vi "query_parts.vi"(8 "error in (no error)":errorcluster, 11 "DB Session ID":i32) -> (0 "error out":errorcluster, 1 "Parts":T1[](array[typedef]), 3 "DB Session ID out":i32)   [LabVIEW 2023, in "Database.lvlib"]
uses:
  Database.lvlib
  DB Part.ctl
  bin/Database.dll
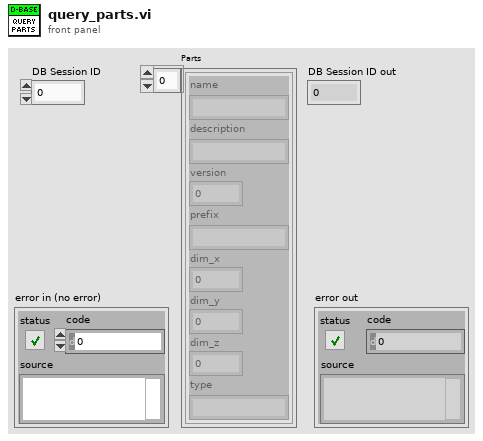
[diagram p1: front panel]
types:
  T1 = typedef "Database.lvlib/DB Part.ctl" = cluster{"name":string, "description":string, "version":i32, "prefix":string, "dim_x":sgl, "dim_y":sgl, "dim_z":sgl, "type":string}
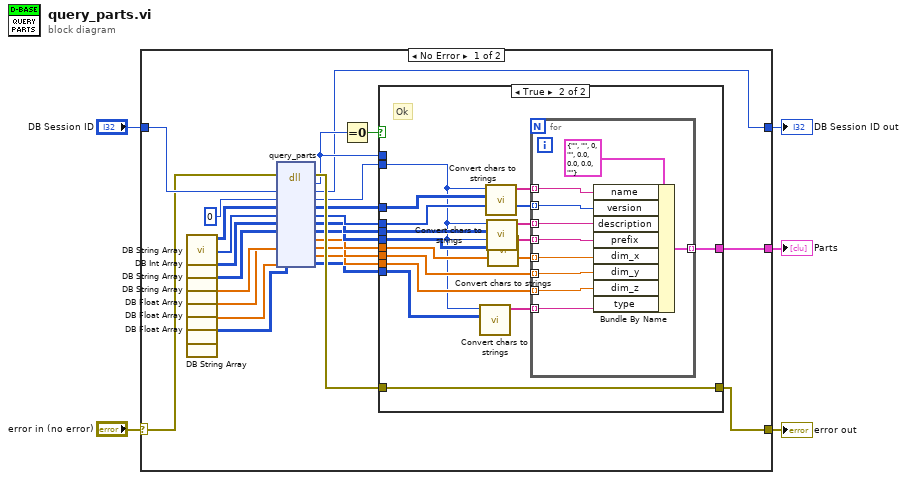
[diagram p0: block diagram]
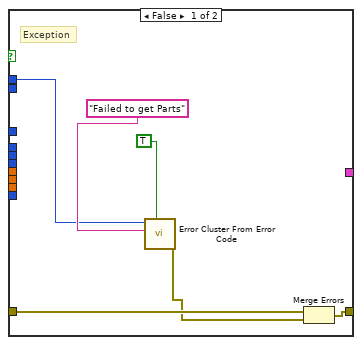
[diagram p2: hidden frame]
diagram:
  n1 = case shown="No Error" "error in (no error)" {
    selector: "error in (no error)" -> [w29 w64]
    tunnel: [w28 w64] -> w3
    tunnel: "DB Session ID" -> [w30 w63]
    tunnel: [w25 _] -> w1
    tunnel: [w23 w63] -> w2
    frame No Error {
      n2 = call "DB String Array.vi"() -> ("DB string array"=w19:i8[][])  [unwired: 11 in]
      n3 = call "DB Int Array.vi"() -> ("DB Int Array"=w18:i32[])  [unwired: 11 in]
      n4 = call "DB String Array.vi"() -> ("DB string array"=w17:i8[][])  [unwired: 11 in]
      n5 = call "DB String Array.vi"() -> ("DB string array"=w16:i8[][])  [unwired: 11 in]
      n6 = call "DB Float Array.vi"() -> ("DB Int Array"=w15:sgl[])  [unwired: 11 in]
      n7 = call "DB Float Array.vi"() -> ("DB Int Array"=w14:sgl[])  [unwired: 11 in]
      n8 = call "DB Float Array.vi"() -> ("DB Int Array"=w13:sgl[])  [unwired: 11 in]
      n9 = call "DB String Array.vi"() -> ("DB string array"=w12:i8[][])  [unwired: 11 in]
      n10 = dll-call lib="C:/Users/cfangmeier3/Desktop/nebraska-silicon-lab/pixel-gantry-control/Gantry/Shared Components/bin/Database.dll" fn="query_parts"(error in=w29, "session_id"=w30, "n_parts"=0, "part"=w19, "version"=w18, "description"=w17, "prefix"=w16, "dim_x"=w15, "dim_y"=w14, "dim_z"=w13, "type"=w12) -> (error out=w31:errorcluster, "return type"=w24:i32, "session_id"=w23:i32, "n_parts"=w20:i32, "part"=w26:i8[][], "version"=w21:i32[], "description"=w11:i8[][], "prefix"=w10:i8[][], "dim_x"=w9:sgl[], "dim_y"=w8:sgl[], "dim_z"=w7:sgl[], "type"=w6:i8[][])  [unwired: 2 in, 1 out]
      n11 = Equal To 0?(x=w24) -> (x = 0?=w27:bool)
      n12 = case shown="True" w27 {
        tunnel: w31 -> [w37 w52]
        tunnel: [w36 w52] -> w28
        tunnel: w26 -> [_ w51]
        tunnel: [_ w49] -> w25
        tunnel: w24 -> [w32 _]
        tunnel: w21 -> [_ w48]
        tunnel: w20 -> [_ w38]
        tunnel: w11 -> [_ w47]
        tunnel: w10 -> [_ w45]
        tunnel: w9 -> [_ w43]
        tunnel: w8 -> [_ w42]
        tunnel: w7 -> [_ w41]
        tunnel: w6 -> [_ w40]
        frame False {
          # "Exception"
          n13 = call <vilib>:"Error Cluster From Error Code.vi"("show call chain? (False)"=TRUE, "error message (\"\")"="Failed to get Parts" ("error message (\"\")"), "error code (0)"=w32) -> ("error out"=w35:errorcluster)  [unwired: 6 in]
          n14 = Merge Errors(w37, w35) -> (w36:errorcluster)
        }
        frame True {
          # "Ok"
          n15 = call "Convert chars to strings.vi"("Char Array"=w40, "Array Length"=w38) -> ("Strings"=w39:string[])  [unwired: 9 in]
          n16 = call "Convert chars to strings.vi"("Char Array"=w51, "Array Length"=w38) -> ("Strings"=w50:string[])  [unwired: 9 in]
          n17 = call "Convert chars to strings.vi"("Char Array"=w47, "Array Length"=w38) -> ("Strings"=w46:string[])  [unwired: 9 in]
          n18 = call "Convert chars to strings.vi"("Char Array"=w45, "Array Length"=w38) -> ("Strings"=w44:string[])  [unwired: 9 in]
          n19 = for {
            tunnel: w50 -> [w60] mode=indexing
            tunnel: [w61] -> w49 mode=indexing
            tunnel: w48 -> [w59] mode=indexing
            tunnel: w46 -> [w58] mode=indexing
            tunnel: w44 -> [w57] mode=indexing
            tunnel: w43 -> [w56] mode=indexing
            tunnel: w42 -> [w55] mode=indexing
            tunnel: w41 -> [w54] mode=indexing
            tunnel: w39 -> [w53] mode=indexing
            n20 = Bundle By Name(cluster=T1 {"name"="", "description"="", "version"=0, "prefix"="", "dim_x"=0.0, "dim_y"=0.0, "dim_z"=0.0, "type"=""} ("Cluster"), "name"=w60, "version"=w59, "description"=w58, "prefix"=w57, "dim_x"=w56, "dim_y"=w55, "dim_z"=w54, "type"=w53) -> (w61:T1)
          }
        }
      }
    }
    frame Error {
    }
  }
  "error out" <- w3
  "DB Session ID out" <- w2
  "Parts" <- w1
